vi "networkCheck.vi"() -> (0 "error out":errorcluster, 1 "standard output":string, 2 "standard error":string, 3 "return code":i32, 4 "T button?":bool)   [LabVIEW 2018, in "wetterLib.lvlib"]
uses:
  wetterLib.lvlib
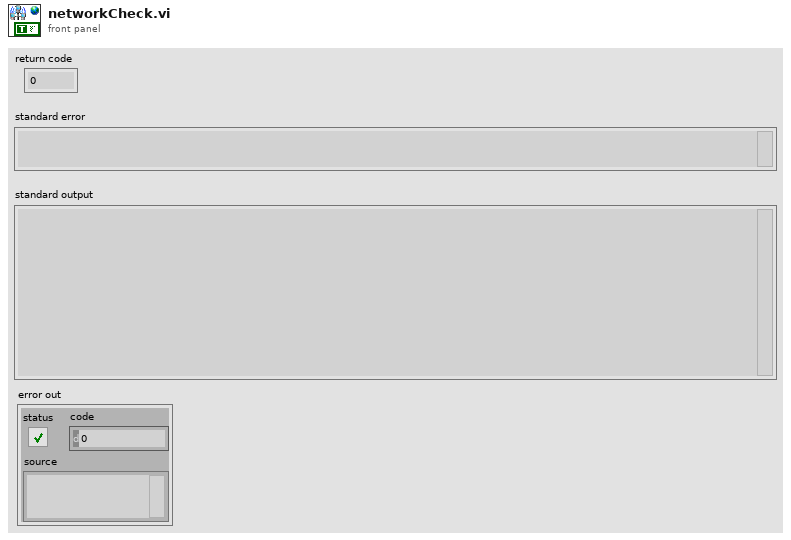
[diagram p1: front panel]
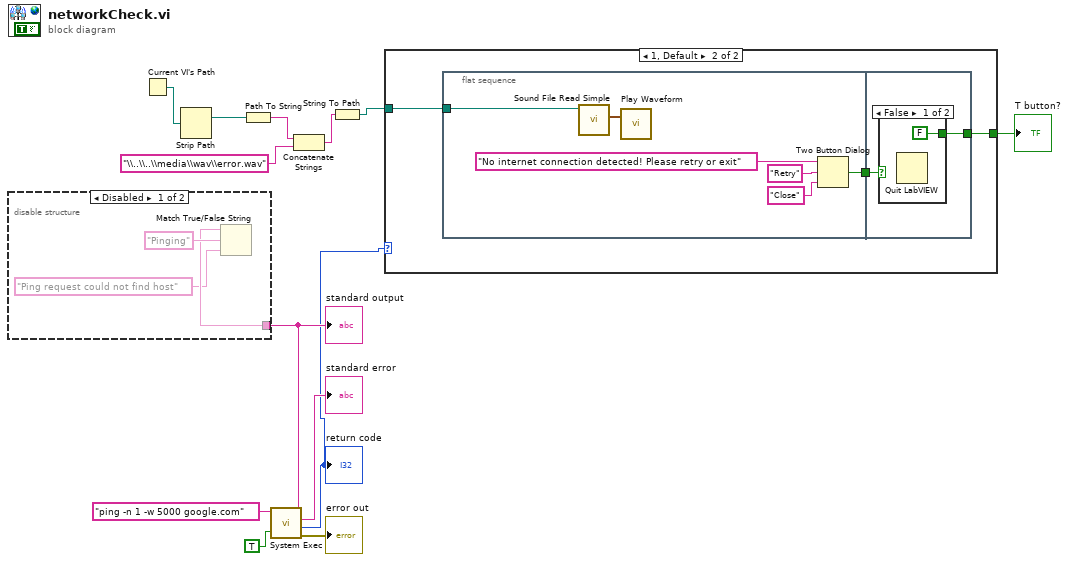
[diagram p0: block diagram]
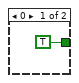
[diagram p3: hidden frame]
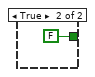
[diagram p4: hidden frame]
diagram:
  n1 = Current VI's Path() -> (path=w7:path)
  n2 = Strip Path(path=w7) -> (stripped path=w6:path)  [unwired: 1 out]
  n3 = Path To String(path=w6) -> (string=w4:string)
  n4 = call <vilib>:"System Exec.vi"("run minimized? (F)"=TRUE, "command line"="ping -n 1 -w 5000 google.com") -> ("error out"=→"error out":errorcluster, "return code"=w1:i32, "standard error"=→"standard error":string, "standard output"=w13:string)  [unwired: 6 in]
  "return code" <- w1
  "standard output" <- w13
  n5 = disable-structure shown="Disabled" {
    disable-tunnel: w13 -> [w15 _]
    frame Disabled {
      n6 = Match True/False String(2:"Ping request could not find host" ("false string"), 3:"Pinging" ("true string"), 4:w15) -> ()  [unwired: 2 out]
    }
    frame Enabled {
    }
  }
  n7 = Concatenate Strings(w4, "\\..\\..\\media\\wav\\error.wav") -> (w3:string)
  n8 = String To Path(string=w3) -> (path=w2:path)
  n9 = case shown="1, Default" w1 {
    tunnel: [TRUE ("T button?") w20] -> w8
    tunnel: w2 -> [_ w18]
    frame 0 {
    }
    frame 1, Default {
      n10 = flat-sequence {
        tunnel: [w25] -> w19
        tunnel: w18 -> [w21]
        tunnel: [w28] -> w20
        tunnel: w19 -> [w27]
        frame #0 {
          n11 = call <vilib>:"Sound File Read Simple.vi"("path"=w21) -> ("data"=w26:waveform(dbl)[])  [unwired: 7 in, 3 out]
          n12 = call "Play Waveform"("Data"=w26) -> ()  [unwired: 18 in, 1 out]
          n13 = Two Button Dialog(message="No internet connection detected! Please retry or exit", 1:"Close" ("F button name (\"Cancel\")"), 2:"Retry" ("Left Button Text (\"Yes\")")) -> (T button?=w25:bool)
        }
        frame #1 {
          n14 = case shown="False" w27 {
            tunnel: [FALSE FALSE] -> w28
            frame False {
              n15 = Quit LabVIEW() -> ()  [unwired: 1 in]
            }
            frame True {
            }
          }
        }
      }
    }
  }
  "T button?" <- w8
